vi "ex_getChannelTypeAI.vi"(8 "error in (no error)":errorcluster, 10 "DAQmx Global Channel":refnum<k21>, 11 "task out":refnum<k21>) -> (0 "error out":errorcluster, 1 "sub type":i32, 2 "subsubtypes":cluster{"String":string, "Value":i32}[](array[cluster]), 3 "dup task":refnum<k21>, 5 "channel type":string)   [LabVIEW 2020]
uses:
  <resource>/objmgr/daqmx.rc
panel:
  in  "CO.OutputType":i32(ring)=10269 items=["Pulse:Time"=10269, "Pulse:Frequency"=10119, "Pulse:Ticks"=10268]
  in  "CI.MeasType":i32(ring)=10125 items=["Count Edges"=10125, "Frequency"=10179, "Period"=10256, "Pulse Width"=10359, "Semi Period"=10289, "Position:Angular Encoder"=10360, "Position:Linear Encoder"=10361, "Two Edge Separation"=10267, "GPS Timestamp"=10362]
  out "ChanType":i32(ring)=10100 items=["Analog Input"=10100, "Analog Output"=10102, "Digital Input"=10151, "Digital Output"=10153, "Counter Input"=10131, "Counter Output"=10132]
  in  "AO.OutputType":i32(ring)=10322 items=["Voltage"=10322, "Current"=10134]
  in  "AI.MeasType":i32(ring)=10322 items=["Voltage"=10322, "Current"=10134, "More:Voltage:Custom with Excitation"=10323, "Frequency"=10181, "Resistance"=10278, "Temperature:Thermocouple"=10303, "Temperature:Thermistor"=10302, "Temperature:RTD"=10301, "Temperature:Built-in Sensor"=10311, "Strain Gage"=10300, "Position:LVDT"=10352, "Position:RVDT"=10353, "Accelerometer"=10356, "Sound Pressure:Microphone"=10354, "TEDS Sensor"=12531]
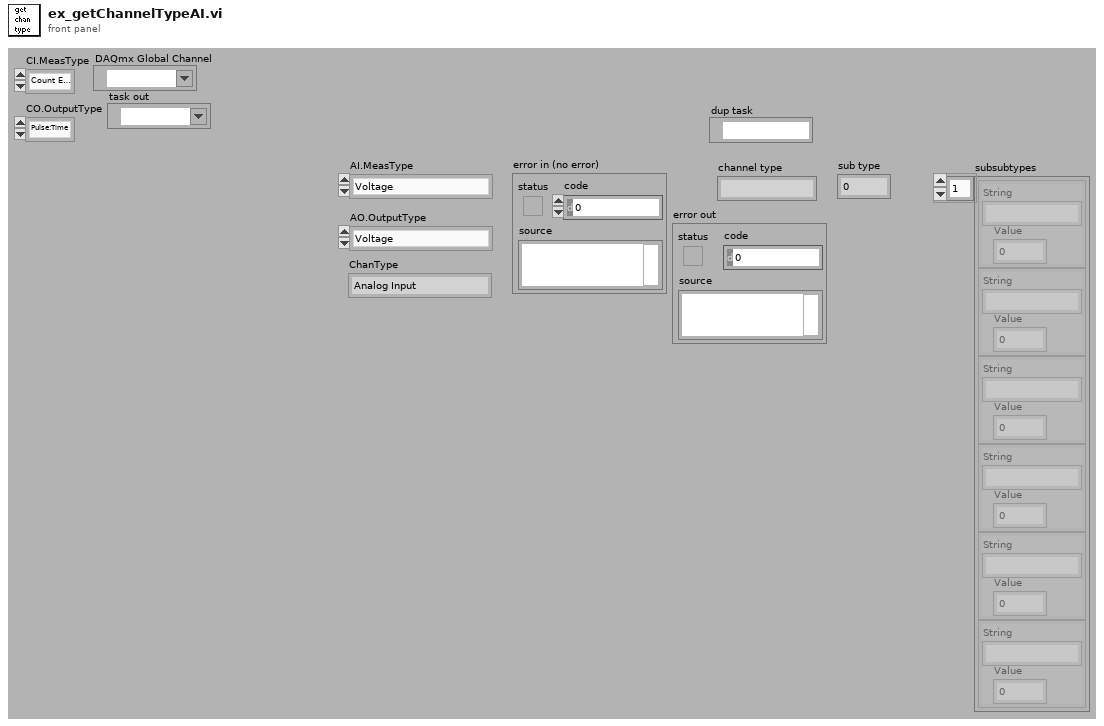
[diagram p1: front panel]
types:
  T1 = typedef "LVStringsAndValuesArrayTypeDef_I32.ctl" = cluster{"String":string, "Value":i32}[]
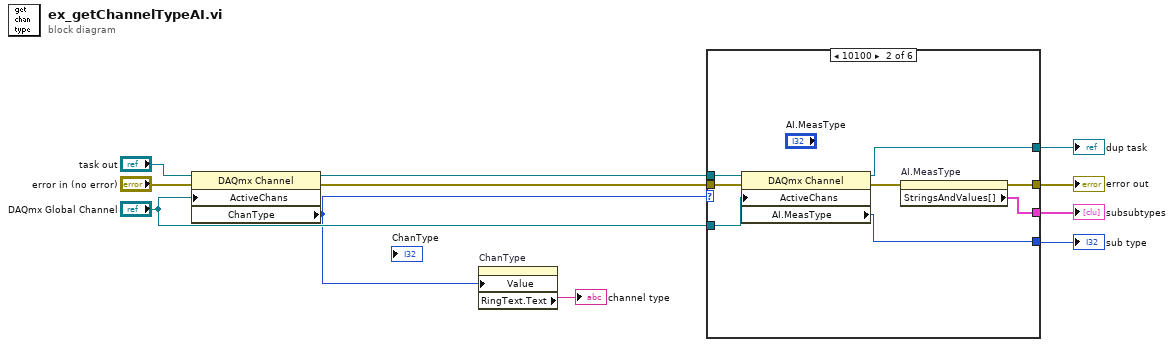
[diagram p0: block diagram]
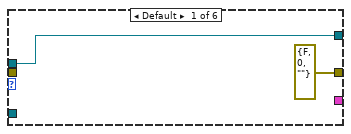
[diagram p2: hidden frame]
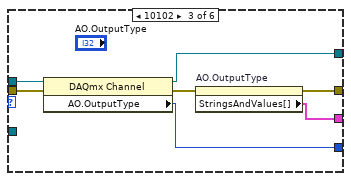
[diagram p3: hidden frame]
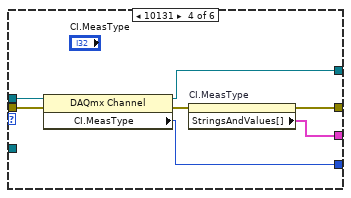
[diagram p4: hidden frame]
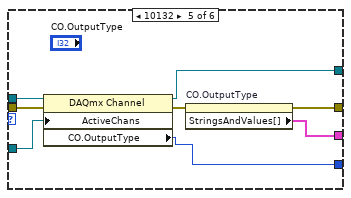
[diagram p5: hidden frame]
diagram:
  n1 = property class="DAQmx Channel"(reference="task out", error in="error in (no error)", "ActiveChans"="DAQmx Global Channel") -> (reference out=w6:refnum<k21>, error out=w7:errorcluster, "ChanType"=w1:i32)
  n2 = property on="ChanType" class="Ring (strict)"("Value"=w1) -> ("RingText.Text"=→"channel type":string)  [unwired: 2 in, 2 out]
  n3 = case shown="10100" w1 {
    tunnel: w7 -> [_ w21 w28 w35 w43 w45]
    tunnel: w6 -> [w13 w20 w27 w34 w42 w44]
    tunnel: [_ w15 w26 w33 w37 _] -> w11
    tunnel: [_ w19 w22 w29 w38 _] -> w10
    tunnel: [w13 w17 w25 w32 w41 w44] -> w9
    tunnel: [errorcluster {"status"=FALSE, "code"=0, "source"=""} ("error out") w16 w23 w30 w39 w45] -> w5
    tunnel: "DAQmx Global Channel" -> [_ w14 _ _ w36 _]
    frame Default {
    }
    frame 10100 {
      n4 = property class="DAQmx Channel"(reference=w20, error in=w21, "ActiveChans"=w14) -> (reference out=w17:refnum<k21>, error out=w18:errorcluster, "AI.MeasType"=w15:i32)
      n5 = property on="AI.MeasType" class="Ring (strict)"(error in=w18) -> (error out=w16:errorcluster, "StringsAndValues[]"=w19:T1)  [unwired: 1 in, 1 out]
    }
    frame 10102 {
      n6 = property class="DAQmx Channel"(reference=w27, error in=w28) -> (reference out=w25:refnum<k21>, error out=w24:errorcluster, "AO.OutputType"=w26:i32)
      n7 = property on="AO.OutputType" class="Ring (strict)"(error in=w24) -> (error out=w23:errorcluster, "StringsAndValues[]"=w22:T1)  [unwired: 1 in, 1 out]
    }
    frame 10131 {
      n8 = property class="DAQmx Channel"(reference=w34, error in=w35) -> (reference out=w32:refnum<k21>, error out=w31:errorcluster, "CI.MeasType"=w33:i32)
      n9 = property on="CI.MeasType" class="Ring (strict)"(error in=w31) -> (error out=w30:errorcluster, "StringsAndValues[]"=w29:T1)  [unwired: 1 in, 1 out]
    }
    frame 10132 {
      n10 = property class="DAQmx Channel"(reference=w42, error in=w43, "ActiveChans"=w36) -> (reference out=w41:refnum<k21>, error out=w40:errorcluster, "CO.OutputType"=w37:i32)
      n11 = property on="CO.OutputType" class="Ring (strict)"(error in=w40) -> (error out=w39:errorcluster, "StringsAndValues[]"=w38:T1)  [unwired: 1 in, 1 out]
    }
    frame 10151, 10153 {
    }
  }
  "sub type" <- w11
  "subsubtypes" <- w10
  "error out" <- w5
  "dup task" <- w9
